vi "Delete Previous gRPC _server and _client Folder.vi"(8 "error in":errorcluster caption="error out", 11 "Template Project Path":path) -> (0 "error out":errorcluster)   [LabVIEW 2021, in "Plugin Generator.lvlib"]
uses:
  Plugin Generator.lvlib
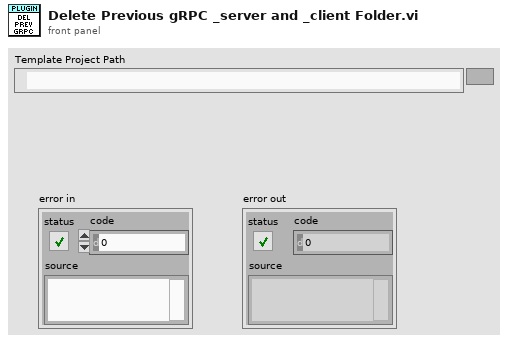
[diagram p1: front panel]
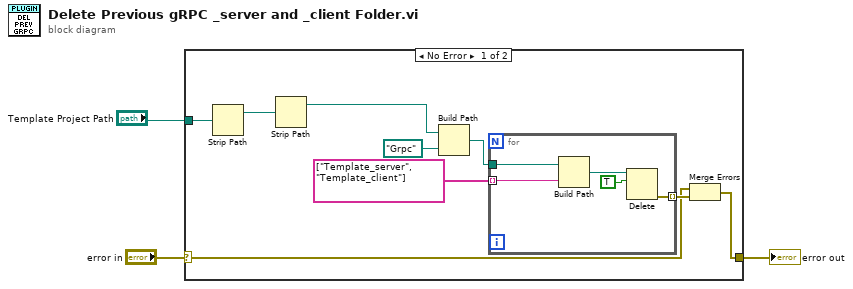
[diagram p0: block diagram]
diagram:
  n1 = case shown="No Error" "error in" {
    selector: "error in" -> [w7 w18]
    tunnel: [w8 w18] -> w2
    tunnel: "Template Project Path" -> [w6 _]
    frame No Error {
      n2 = Strip Path(path=w6) -> (stripped path=w5:path)  [unwired: 1 out]
      n3 = Strip Path(path=w5) -> (stripped path=w4:path)  [unwired: 1 out]
      n4 = Build Path(base path=w4, name or relative path=path "Grpc") -> (appended path=w10:path)
      n5 = for {
        tunnel: [w17] -> w9 mode=indexing
        tunnel: w10 -> [w15]
        tunnel: string[] ["Template_server", "Template_client"] -> [w13] mode=indexing
        n6 = Build Path(base path=w15, name or relative path=w13) -> (appended path=w14:path)
        n7 = Delete(path (use dialog)=w14, entire hierarchy (F)=TRUE) -> (error out=w17:errorcluster)  [unwired: 3 in, 2 out]
      }
      n8 = Merge Errors(w7, w9) -> (w8:errorcluster)
    }
    frame Error {
    }
  }
  "error out" <- w2
